vi "WriteToBaseConfigVariant.vi"(6 "Measurement Refresh Time (ms)":u32, 8 "error in (no error)":errorcluster, 9 "Meas":variant, 10 "Config":variant, 11 "ChromaPowerSupplyModel in":refnum<class "ChromaPowerSupplyModel.lvclass">) -> (0 "error out":errorcluster, 3 "ChromaPowerSupplyModel out":refnum<class "ChromaPowerSupplyModel.lvclass">)   [LabVIEW 2018, in "AcPwrPlugins.lvlib" / "ChromaPowerSupplyModel.lvclass"]
uses:
  ChromaPowerSupplyModel.lvclass
  C:/Projects/SmartGrid/ICDAS/NistPluggableModules/AcPwr/AcPwrPlugins/AcPwrBaseClass/AcPwrBase.lvclass
  AcPwrBaseClass/AcPwrBase.lvclass/AcPwrBase.ctl
  AcPwrBaseClass/Accessors/Read BaseConfig.vi
  AcPwrBaseClass/Accessors/Write BaseConfig.vi
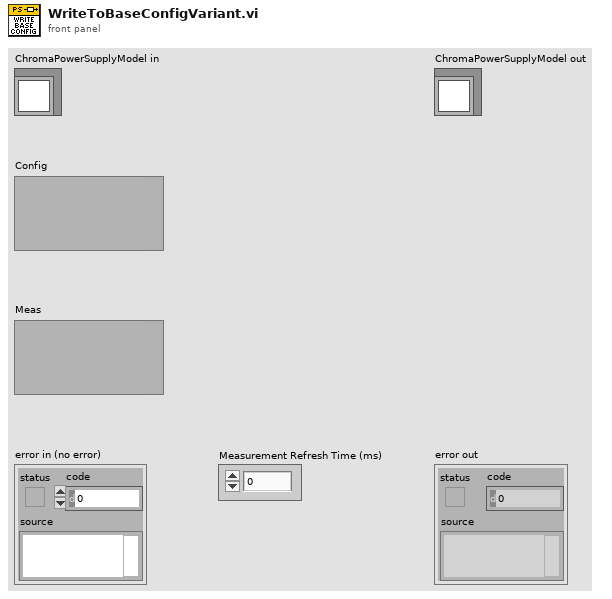
[diagram p1: front panel]
types:
  T1 = typedef "AcPwrPlugins.lvlib/AcPwrBase.lvclass/BaseConfig.ctl" = cluster{"Frequency":dbl, "FrequencyRange":dbl[], "Phases":T2[], "Name":string, "PluginConfigVariant":variant, "PluginMeasVariant":variant}
  T2 = typedef "AcPwrPlugins.lvlib/AcPwrBase.lvclass/Phase.ctl" = cluster{"Name":string, "Enabled":bool, "VoltageLevel":dbl, "Handle":string, "VoltageRange":dbl[], "Connected":bool, "CurrentLimit":dbl, "Waveform":string}
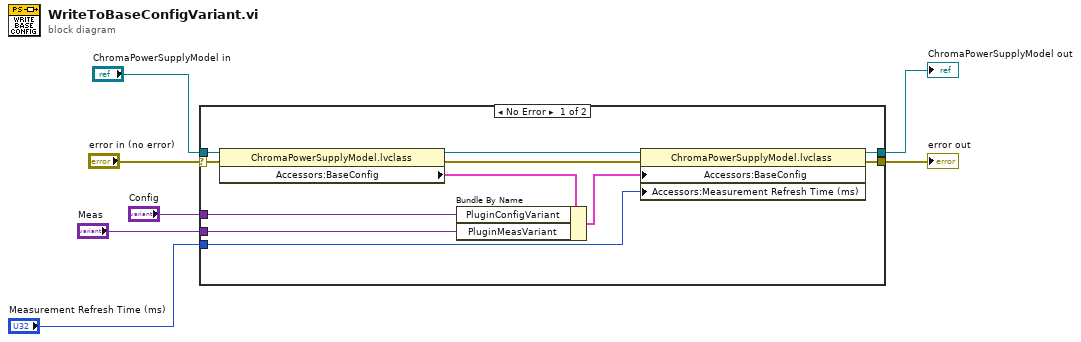
[diagram p0: block diagram]
diagram:
  n1 = case shown="No Error" "error in (no error)" {
    selector: "error in (no error)" -> [w18 w20]
    tunnel: [w14 w20] -> w1
    tunnel: [w13 w19] -> w6
    tunnel: "ChromaPowerSupplyModel in" -> [w8 w19]
    tunnel: "Config" -> [w15 _]
    tunnel: "Meas" -> [w11 _]
    tunnel: "Measurement Refresh Time (ms)" -> [w10 _]
    frame No Error {
      n2 = property class="ChromaPowerSupplyModel.lvclass"(reference=w8, error in=w18) -> (reference out=w9:refnum<class "ChromaPowerSupplyModel.lvclass">, error out=w17:errorcluster, "Accessors:BaseConfig"=w16:T1)
      n3 = Bundle By Name(cluster=w16, "PluginConfigVariant"=w15, "PluginMeasVariant"=w11) -> (w12:T1)
      n4 = property class="ChromaPowerSupplyModel.lvclass"(reference=w9, error in=w17, "Accessors:BaseConfig"=w12, "Accessors:Measurement Refresh Time (ms)"=w10) -> (reference out=w13:refnum<class "ChromaPowerSupplyModel.lvclass">, error out=w14:errorcluster)
    }
    frame Error {
    }
  }
  "error out" <- w1
  "ChromaPowerSupplyModel out" <- w6
